vi "Update.vi"(8 "error in (no error)":errorcluster, 10 "Message in":refnum<class "UpdateMessage.lvclass">, 11 "ServiceManager in":refnum<class "ServiceManager.lvclass">) -> (0 "error out":errorcluster, 3 "ServiceManager out":refnum<class "ServiceManager.lvclass">)   [LabVIEW 2012, in "ServiceManager.lvclass"]
doc: "The update method processes the command 'update'. \n\nThe command 'update' is used for receiving new values to be set to the private data of the class. This could be seen as a public set method for setting new parameters to the private class data."
uses:
  ServiceManager.lvclass
  Murmex/LabVIEW/Murmex/UpdateMessage/UpdateMessage.lvclass
  Murmex/LabVIEW/Murmex/Murmex/Murmex.lvclass
  ServiceManager.lvclass/ServiceManager.ctl
panel:
  # "This method is called when the UPDATE\ntrigger is sent. \n\nOverride this method when your component needs to\nrespond to this trigger. \n\nCall parent for proper implementation"
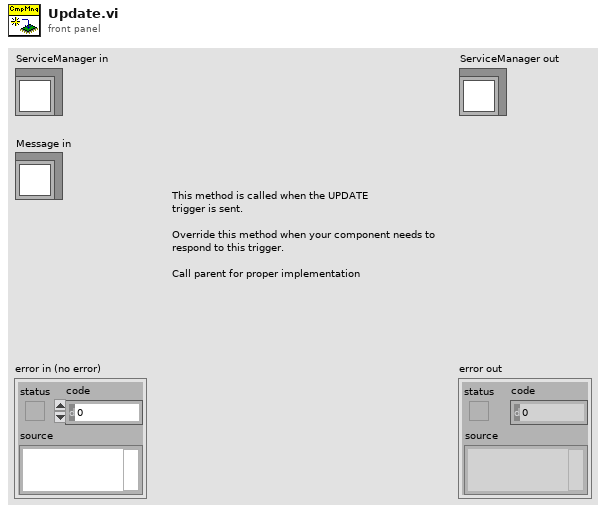
[diagram p1: front panel]
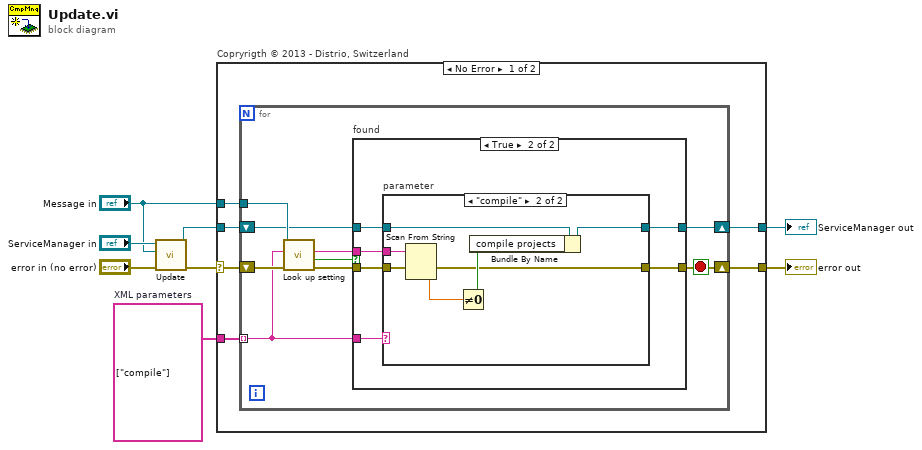
[diagram p0: block diagram]
diagram:
  w4 = string[] ["compile"]  # XML parameters
  n1 = call-parent "Update.vi"("error in (no error)"="error in (no error)", "Message in"="Message in", "Murmex in"="ServiceManager in") -> ("error out"=w6:errorcluster, "Murmex out"=w5:refnum<class "ServiceManager.lvclass">)  [unwired: 7 in]
  n2 = case "Copryrigth © 2013 - Distrio, Switzerland" shown="No Error" w6 {
    selector: w6 -> [w14 w41]
    tunnel: w5 -> [w11 w42]
    tunnel: w4 -> [w12 _]
    tunnel: "Message in" -> [w13 _]
    tunnel: [w10 w41] -> w3
    tunnel: [w9 w42] -> w2
    frame No Error {
      n3 = for {
        tunnel: w13 -> [w22]
        tunnel: w12 -> [w19] mode=indexing
        shift-right: [w15] -> w10
        shift-left: w14 -> [w23]
        shift-right: [w16] -> w9
        shift-left: w11 -> [w17]
        stop <- w15 stop-if-true
        n4 = call "Look up setting.vi"("error in (no error)"=w23, "tag name"=w19, "UpdateMessage in"=w22) -> ("error out"=w18:errorcluster, "found?"=w21:bool, "value"=w20:string)  [unwired: 5 in, 1 out]
        n5 = case "found" shown="True" w21 {
          tunnel: w20 -> [_ w28]
          tunnel: w19 -> [_ w31]
          tunnel: w18 -> [w24 w30]
          tunnel: w17 -> [w25 w29]
          tunnel: [w24 w27] -> w15
          tunnel: [w25 w26] -> w16
          frame False {
          }
          frame True {
            n6 = case "parameter" shown="\"compile\"" w31 {
              tunnel: w30 -> [w32 w39]
              tunnel: w29 -> [w33 w40]
              tunnel: w28 -> [_ w38]
              tunnel: [w32 w35] -> w27
              tunnel: [w33 w34] -> w26
              frame Default {
              }
              frame "compile" {
                n7 = Scan From String(input string=w38, error in=w39) -> (error out=w35:errorcluster, output 1=w37:dbl)  [unwired: 3 in, 2 out]
                n8 = Not Equal To 0?(x=w37) -> (x != 0?=w36:bool)
                n9 = Bundle By Name(cluster=w40, "compile projects"=w36) -> (w34:refnum<class "ServiceManager.lvclass">)
              }
            }
          }
        }
      }
    }
    frame Error {
    }
  }
  "error out" <- w3
  "ServiceManager out" <- w2
